vi "FaultCheck.vi"(8 "error in (no error)":errorcluster, 10 "Cluster in":T2, 11 "Enum in":T1) -> (0 "error out":errorcluster, 2 "Cluster out":T2, 3 "Enum out":T1)   [LabVIEW 2018]
uses:
  Type_Def/Type_Def Actuator Controls.ctl
  Type_Def/Type_Def ControlState.ctl
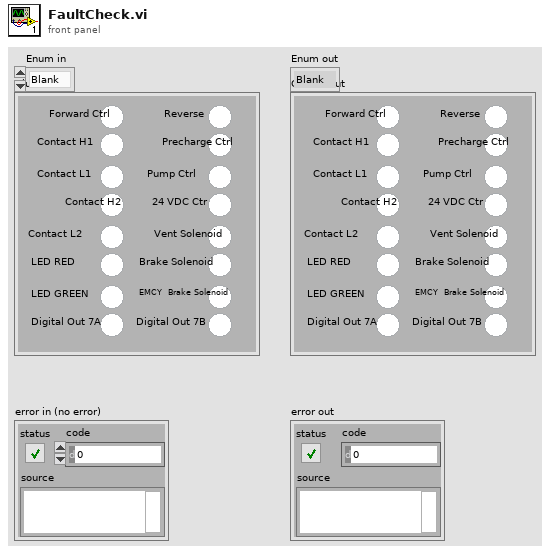
[diagram p1: front panel]
types:
  T1 = typedef "Type_Def ControlState.ctl" = enum16{"Blank", "Systems Check", "Idle", "Ready", "Pushing", "CrawlingPrecharge", "Braking", "Fault", "Boot Up", "Unpowered", "Crawling", "Shutdown", "Service Push", "Service Wait", "Vent", "Precharge"}
  T2 = typedef "Type_Def Actuator Controls.ctl" = cluster{"Reverse ":bool, "Precharge Ctrl":bool, "Pump Ctrl":bool, "24 VDC Ctr":bool, "Vent Solenoid":bool, "Brake Solenoid":bool, "EMCY  Brake Solenoid":bool, "Digital Out 7B ":bool, "Forward Ctrl":bool, "Contact H1":bool, "Contact L1":bool, "Contact H2":bool, "Contact L2 ":bool, "LED RED":bool, "LED GREEN":bool, " Digital Out 7A":bool}
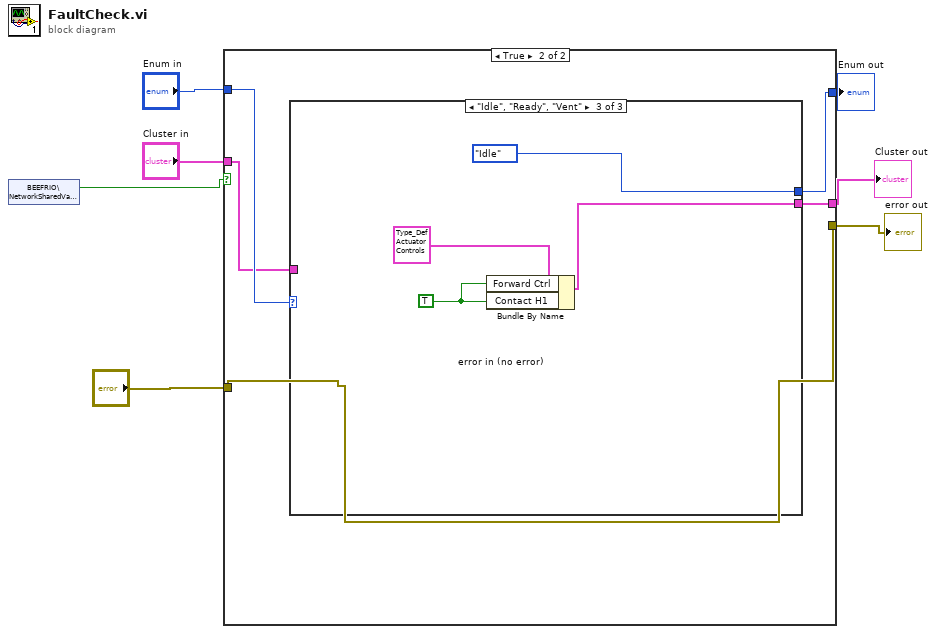
[diagram p0: block diagram]
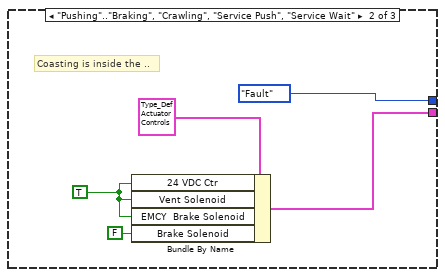
[diagram p4: hidden frame]
diagram:
  n1 = shared-variable "BEEFRIO\\NetworkSharedVariable.lvlib\\Fault"() -> (w1:bool)  [unwired: 1 in, 1 out]
  n2 = case shown="True" w1 {
    tunnel: [w10 w11] -> w7
    tunnel: "error in (no error)" -> [w10 w11]
    tunnel: [w9 w13] -> w5
    tunnel: "Cluster in" -> [w9 w12]
    tunnel: [w8 w14] -> w3
    tunnel: "Enum in" -> [w8 w15]
    frame False {
    }
    frame True {
      n3 = case shown="\"Idle\", \"Ready\", \"Vent\"" w15 {
        selector: w15 -> [w16 _ _]
        tunnel: [w16 Type_Def_ControlState."Fault" ("Enum in 2") Type_Def_ControlState."Idle" ("Enum in 2")] -> w14
        tunnel: [w17 w21 w25] -> w13
        tunnel: w12 -> [w17 _ _]
        frame Default {
        }
        frame "Pushing".."Braking", "Crawling", "Service Push", "Service Wait" {
          w19 = TRUE
          # "Coasting is inside the .."
          n4 = Bundle By Name(cluster=T2 {"Reverse "=FALSE, "Precharge Ctrl"=FALSE, "Pump Ctrl"=FALSE, "24 VDC Ctr"=FALSE, "Vent Solenoid"=FALSE, "Brake Solenoid"=FALSE, "EMCY  Brake Solenoid"=FALSE, "Digital Out 7B "=FALSE, "Forward Ctrl"=FALSE, "Contact H1"=FALSE, "Contact L1"=FALSE, "Contact H2"=FALSE, "Contact L2 "=FALSE, "LED RED"=FALSE, "LED GREEN"=FALSE, " Digital Out 7A"=FALSE} ("Cluster in 2"), "24 VDC Ctr"=w19, "Vent Solenoid"=w19, "EMCY  Brake Solenoid"=w19, "Brake Solenoid"=FALSE ("EMCY  Brake Solenoid")) -> (w21:T2)
        }
        frame "Idle", "Ready", "Vent" {
          w23 = TRUE
          n5 = Bundle By Name(cluster=T2 {"Reverse "=FALSE, "Precharge Ctrl"=FALSE, "Pump Ctrl"=FALSE, "24 VDC Ctr"=FALSE, "Vent Solenoid"=FALSE, "Brake Solenoid"=FALSE, "EMCY  Brake Solenoid"=FALSE, "Digital Out 7B "=FALSE, "Forward Ctrl"=FALSE, "Contact H1"=FALSE, "Contact L1"=FALSE, "Contact H2"=FALSE, "Contact L2 "=FALSE, "LED RED"=FALSE, "LED GREEN"=FALSE, " Digital Out 7A"=FALSE} ("Cluster in 2"), "Forward Ctrl"=w23, "Contact H1"=w23) -> (w25:T2)
        }
      }
    }
  }
  "error out" <- w7
  "Cluster out" <- w5
  "Enum out" <- w3
